vi "Get-Version.vi"() -> (3 "Version":string="1.0.0")   [LabVIEW 2017]
uses:
  Globals.vi
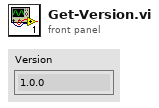
[diagram p1: front panel]
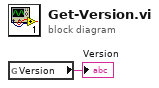
[diagram p0: block diagram]
diagram:
  n1 = global read "Globals.vi" "Version"() -> (→"Version":string)
